vi "Check If Receiver Is Local.vi"(0 "message":T1, 5 "UDP receiver port":u16, 11 "error in":errorcluster) -> (4 "local receiver?":bool, 15 "error out":errorcluster)   [LabVIEW 2014, in "AMC.lvlib"]
doc: "Check if the receiver specified in the message is the same as the local application.\n\nThe receiver is considered local if:\n-\"receiver host\" or \"receiver process\" is empty.\nor\n-\"receiver host\" matches the local IP address and \"UDP reciever port\" matches the local UDP Dispatcher port."
uses:
  AMC.lvlib
  Message.ctl
  <vilib>/NI/Tools/Keyed Array/KeyedArray.ctl
  <vilib>/NI/Tools/Keyed Array/Tools_KeyedArray.lvlib
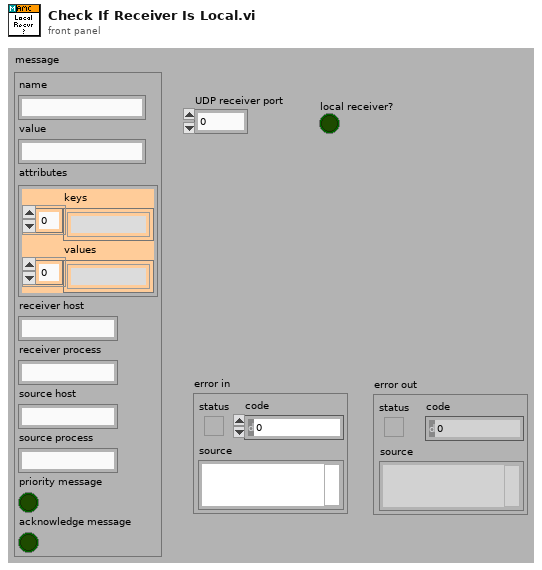
[diagram p1: front panel]
types:
  T1 = typedef "AMC.lvlib/Message.ctl" = cluster{"name":string, "value":string, "attributes":T2, "receiver host":string, "receiver process":string, "source host":string, "source process":string, "priority message":bool, "acknowledge message":bool}
  T2 = typedef "Tools_KeyedArray.lvlib/KeyedArray.ctl" = cluster{"keys":string[], "values":string[]}
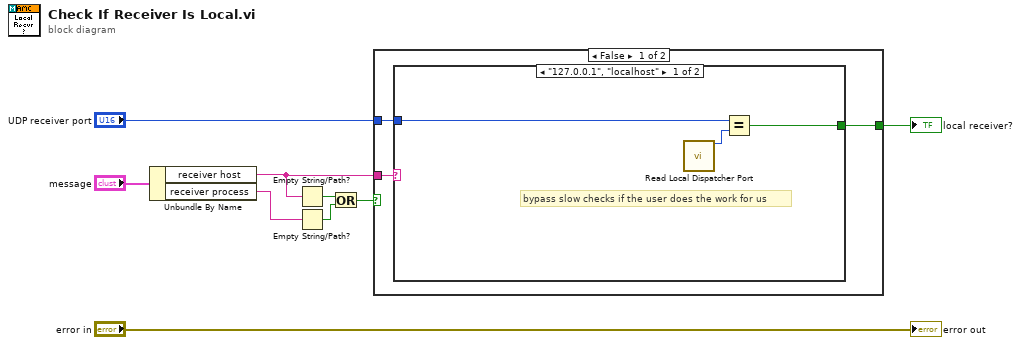
[diagram p0: block diagram]
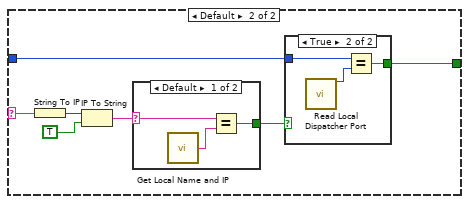
[diagram p2: hidden frame]
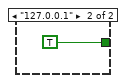
[diagram p4: hidden frame]
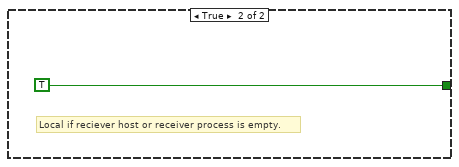
[diagram p5: hidden frame]
diagram:
  n1 = Unbundle By Name("message") -> ("receiver host"=w4:string, "receiver process"=w3:string)
  n2 = Empty String/Path?(string/path=w4) -> (empty?=w6:bool)
  n3 = Empty String/Path?(string/path=w3) -> (empty?=w7:bool)
  n4 = Or(x=w6, y=w7) -> (x .or. y?=w5:bool)
  n5 = case shown="False" w5 {
    tunnel: w4 -> [w10 _]
    tunnel: [w11 TRUE] -> w2
    tunnel: "UDP receiver port" -> [w12 _]
    frame False {
      n6 = case shown="\"127.0.0.1\", \"localhost\"" w10 {
        selector: w10 -> [_ w16]
        tunnel: w12 -> [w14 w18]
        tunnel: [w13 w17] -> w11
        frame "127.0.0.1", "localhost" {
          # "bypass slow checks if the user does the work for us"
          n7 = call "Read Local Dispatcher Port.vi"() -> ("UDP port"=w15:u16)  [unwired: 14 in, 1 out]
          n8 = Equal?(x=w14, y=w15) -> (x = y?=w13:bool)
        }
        frame Default {
          n9 = String To IP(1:w16) -> (0:w21:u32)
          n10 = IP To String(1:TRUE ("dot notation? (F)"), 2:w21) -> (0:w20:string)
          n11 = case shown="Default" w20 {
            selector: w20 -> [w28 _]
            tunnel: [w27 TRUE] -> w19
            frame Default {
              n12 = call "Get Local Name and IP.vi"() -> ("IP address"=w26:string)  [unwired: 12 in, 3 out]
              n13 = Equal?(x=w28, y=w26) -> (x = y?=w27:bool)
            }
            frame "127.0.0.1" {
            }
          }
          n14 = case shown="True" w19 {
            tunnel: w18 -> [_ w25]
            tunnel: [_ w23] -> w17
            frame False {
            }
            frame True {
              n15 = call "Read Local Dispatcher Port.vi"() -> ("UDP port"=w24:u16)  [unwired: 14 in, 1 out]
              n16 = Equal?(x=w25, y=w24) -> (x = y?=w23:bool)
            }
          }
        }
      }
    }
    frame True {
      # "Local if reciever host or receiver process is empty."
    }
  }
  "local receiver?" <- w2
  "error out" <- "error in"
